vi "Bit_To_Degree_Conversion.vi"(10 "Actual joints positions":T3(array[cluster]) {"Error Code" format="%b"; "ID" format="%x"}) -> (2 "Motor positions (degree)":T1(array[cluster]) {"Error Code (bits)" format="%b"})   [LabVIEW 2015]
panel:
  in  "Motor info":T2 {"Error Code (bits)" format="%b"}
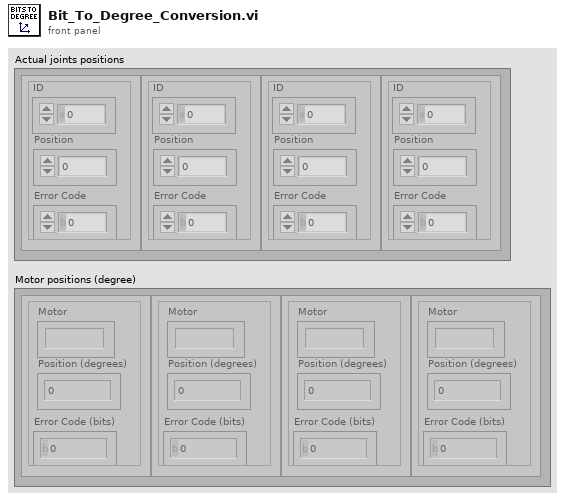
[diagram p1: front panel]
types:
  T1 = cluster{"Position (degrees)":i32, "Error Code (bits)":u8, "Motor":string}[]
  T2 = cluster{"Position (degrees)":i32, "Error Code (bits)":u8, "Motor":string}
  T3 = cluster{"ID":u8, "Position":u16, "Error Code":u8}[]
  T4 = cluster{"ID":u8, "Position":u16, "Error Code":u8}
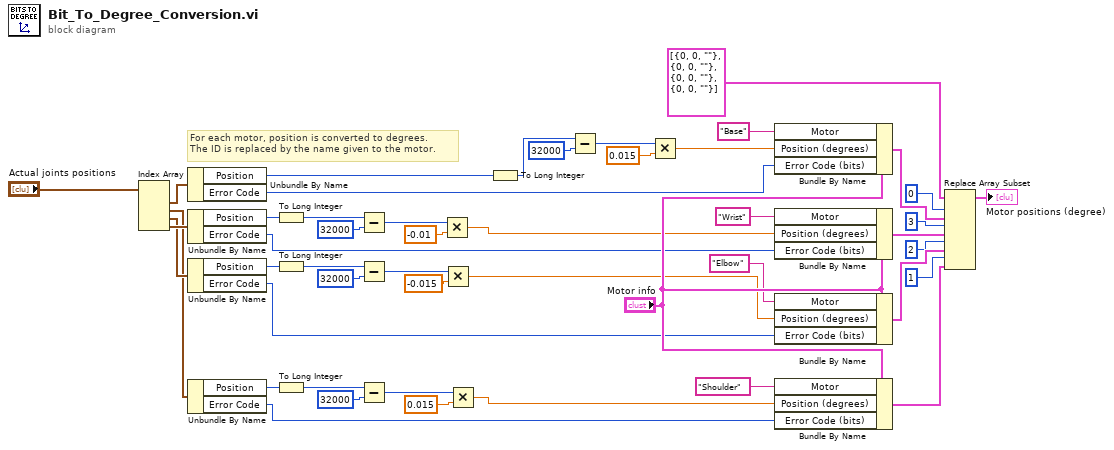
[diagram p0: block diagram]
diagram:
  # "For each motor, position is converted to degrees.\nThe ID is replaced by the name given to the motor."
  n1 = Index Array(array="Actual joints positions") -> (element #1=w24:T4, element #2=w46:T4, element #3=w47:T4, element #4=w48:T4)  [unwired: 4 in]
  n2 = Unbundle By Name(w24) -> ("Position"=w41:u16, "Error Code"=w22:u8)
  n3 = Unbundle By Name(w48) -> ("Position"=w26:u16, "Error Code"=w16:u8)
  n4 = Unbundle By Name(w47) -> ("Position"=w31:u16, "Error Code"=w15:u8)
  n5 = Unbundle By Name(w46) -> ("Position"=w36:u16, "Error Code"=w14:u8)
  n6 = To Long Integer(number=w26) -> (32bit integer=w30:i32)
  n7 = To Long Integer(number=w31) -> (32bit integer=w32:i32)
  n8 = To Long Integer(number=w36) -> (32bit integer=w40:i32)
  n9 = Subtract(x=w30, y=i16 32000) -> (x-y=w28:i32)
  n10 = Subtract(x=w32, y=i16 32000) -> (x-y=w34:i32)
  n11 = Subtract(x=w40, y=i16 32000) -> (x-y=w38:i32)
  n12 = Multiply(x=w28, y=-0.01) -> (x*y=w17:dbl)
  n13 = Multiply(x=w34, y=-0.015) -> (x*y=w18:dbl)
  n14 = Multiply(x=w38, y=0.015) -> (x*y=w19:dbl)
  n15 = To Long Integer(number=w41) -> (32bit integer=w42:i32)
  n16 = Subtract(x=w42, y=i16 32000) -> (x-y=w44:i32)
  n17 = Multiply(x=w44, y=0.015) -> (x*y=w23:dbl)
  n18 = Bundle By Name(cluster="Motor info", "Motor"="Base", "Position (degrees)"=w23, "Error Code (bits)"=w22) -> (w10:T2)
  n19 = Bundle By Name(cluster="Motor info", "Motor"="Wrist", "Position (degrees)"=w17, "Error Code (bits)"=w16) -> (w9:T2)
  n20 = Bundle By Name(cluster="Motor info", "Motor"="Elbow", "Position (degrees)"=w18, "Error Code (bits)"=w15) -> (w8:T2)
  n21 = Bundle By Name(cluster="Motor info", "Motor"="Shoulder", "Position (degrees)"=w19, "Error Code (bits)"=w14) -> (w7:T2)
  n22 = Replace Array Subset(array=T1 [{"Position (degrees)"=0, "Error Code (bits)"=0, "Motor"=""}, {"Position (degrees)"=0, "Error Code (bits)"=0, "Motor"=""}, {"Position (degrees)"=0, "Error Code (bits)"=0, "Motor"=""}, {"Position (degrees)"=0, "Error Code (bits)"=0, "Motor"=""}] ("Actual joints positions (degree)"), new element #1=w10, index #1=0 ("index"), new element #2=w9, index #2=3 ("index"), new element #3=w8, index #3=2 ("index"), new element #4=w7, index #4=1 ("index")) -> (→"Motor positions (degree)":T1)
